vi "Set PWM Enable.vi"(7 "GPIO":i32, 8 "error in (no error)":errorcluster, 10 "Enable":bool, 11 "VISA resource name in":refnum<visa-resource-name>) -> (0 "error out":errorcluster, 3 "VISA resource name":refnum<visa-resource-name>)   [LabVIEW 2020, in "CTI-Visa.lvlib"]
uses:
  CTI-Visa.lvlib
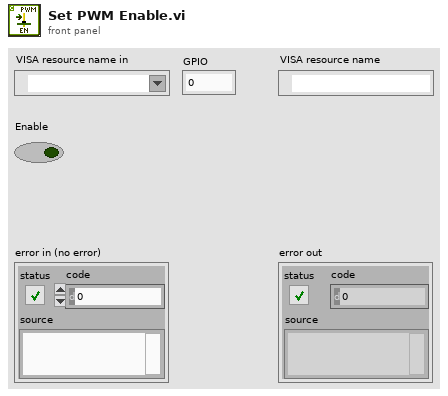
[diagram p1: front panel]
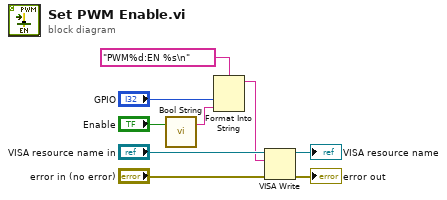
[diagram p0: block diagram]
diagram:
  n1 = call "Bool String.vi"("Bool"="Enable") -> ("String"=w6:string)  [unwired: 6 in]
  n2 = Format Into String(format string="PWM%d:EN %s\n", "GPIO", w6) -> (resulting string=w4:string)  [unwired: 2 in, 1 out]
  n3 = VISA Write(VISA resource name="VISA resource name in", write buffer=w4, error in (no error)="error in (no error)") -> (VISA resource name out=→"VISA resource name":refnum<visa-resource-name>, error out=→"error out":errorcluster)  [unwired: 1 out]
